vi "Drop NotifyIcon.vi"(4 "error in (no error)":errorcluster, 7 "NotifyIcon":refnum<k24>) -> (0 "error out":errorcluster)   [LabVIEW 2020, in "NotifyIcon.lvlib"]
uses:
  NotifyIcon.lvlib
  System.Windows.Forms
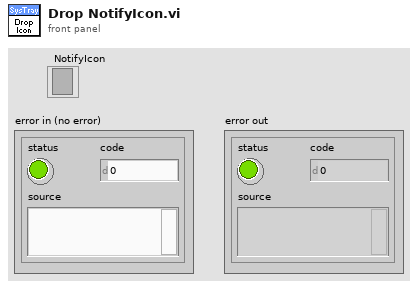
[diagram p1: front panel]
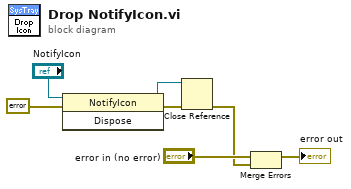
[diagram p0: block diagram]
diagram:
  n1 = invoke class="NotifyIcon" method="Dispose"(reference="NotifyIcon", error in=errorcluster {"status"=FALSE, "code"=0, "source"=""} ("error in (no error)")) -> (reference out=w6:refnum<k24>, error out=w5:errorcluster)  [unwired: 1 in, 1 out]
  n2 = Close Reference(reference=w6, error in (no error)=w5) -> (error out=w2:errorcluster)
  n3 = Merge Errors("error in (no error)", w2) -> (→"error out":errorcluster)
